vi "Choose_USB.vi"() -> (2 "Annulé?":bool, 3 "Nom de ressource VISA en sortie":refnum<visa-resource-name>)   [LabVIEW 2013]
panel:
  in  "Bouton Annuler":bool
  in  "Bouton OK":bool
  in  "Nom de ressource VISA":refnum<visa-resource-name>
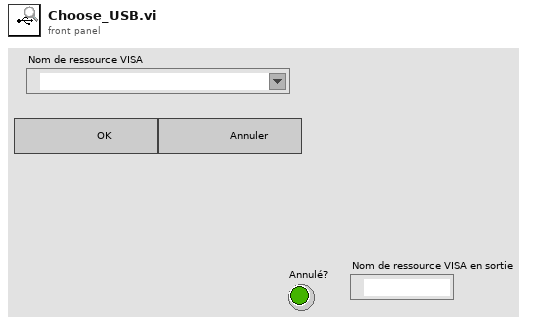
[diagram p1: front panel]
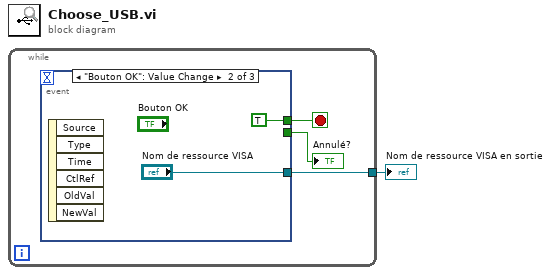
[diagram p0: block diagram]
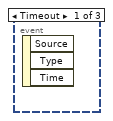
[diagram p2: hidden frame]
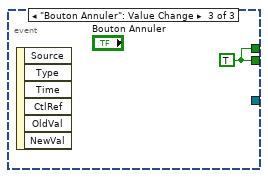
[diagram p3: hidden frame]
diagram:
  n1 = while {
    tunnel: [w2] -> w1
    stop <- w4 stop-if-true
    n2 = event shown="[1] \"Bouton OK\": Value Change" {
      selector: _ -> [_ _ _]
      dyn-events: _ -> [_ _ _]
      timeout: _ -> [_ _ _]
      tunnel: [_ TRUE w7] -> w4
      tunnel: [_ _ w7] -> w3
      tunnel: [_ "Nom de ressource VISA" _] -> w2
      event Timeout {
        n3 = event-data() -> ()  [unwired: 1 in, 3 out]
      }
      event "Bouton OK": Value Change {
        n4 = event-data() -> ()  [unwired: 1 in, 6 out]
      }
      event "Bouton Annuler": Value Change {
        w7 = TRUE
        n5 = event-data() -> ()  [unwired: 1 in, 6 out]
      }
    }
    "Annulé?" <- w3
  }
  "Nom de ressource VISA en sortie" <- w1
